vi "IMA Check Stop DC.vi"(0 "WFDC Notifier":refnum<notifier>, 7 "WFDC External Sync":refnum<notifier>, 11 "Error":errorcluster) -> (4 "WFDC Notifier (Dup)":refnum<notifier>, 8 "WFDC External Sync (Dup)":refnum<notifier>, 15 "Error Out":errorcluster)   [LabVIEW 2020]
uses:
  Wide Field Drift Correction/WFDC Controls/WFDC External Sync.ctl
  Wide Field Drift Correction/WFDC Controls/WFDC Cycle Pause.ctl
  Wide Field Drift Correction/WFDC Controls/WFDC Status.ctl
  Wide Field Drift Correction/WFDC Controls/WFDC Notifier Element.ctl
  Wide Field Drift Correction/WFDC Controls/WFDC Actions.ctl
  <vilib>/vision/Image Controls.llb/IMAQ Image.ctl
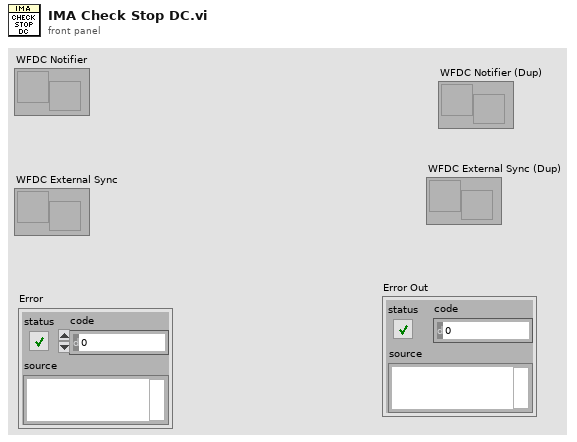
[diagram p1: front panel]
types:
  T1 = typedef "WFDC External Sync.ctl" = cluster{"Cycle Sync":T2, "Z Offset":dbl, "WFDC Status":T3}
  T2 = typedef "WFDC Cycle Pause.ctl" = enum16{"Pause Requested", "Paused", "Resume Requested", "Resumed"}
  T3 = typedef "WFDC Status.ctl" = enum16{"Idle", "Busy", "DC Active", "Error", "Canceled"}
  T4 = typedef "WFDC Notifier Element.ctl" = cluster{"WFDC Actions":T5, "Initial XYZ Positions":dbl[], "Ref Images":T6[], "Calibration (slope, inter)":dbl[], "Base Path":path, "Latest Scan Path":path, "Error":errorcluster, "XYZ Drift":dbl[]}
  T5 = typedef "WFDC Actions.ctl" = enum16{"Error Check", "Remote Start", "Move to Pos", "Pre Start Get Drift", "Pre Start Check Drift", "Pre Start Z Drift", "Pre Start XY Drift", "Pre Start ReFocus", "Setup New DC", "Setup Camera", "Get Ref Images", "Calc Calibration", "Switch Tabs", "Get Drift", "Z Drift", "XY Drift", "Start Cycle", "Stop DC", "Abort Remote", "Exit Loop", "Set Error", "Generate Calibration", "Quit"}
  T6 = typedef "IMAQ Image.ctl" = refnum<image>
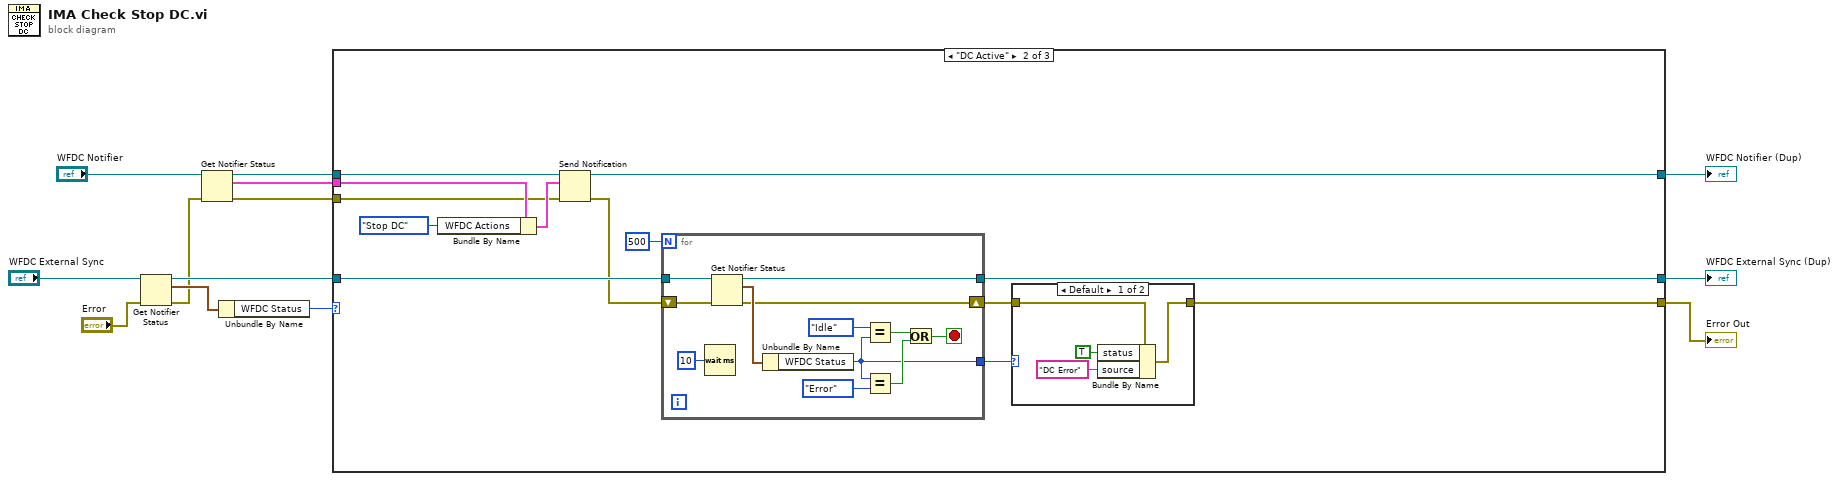
[diagram p0: block diagram]
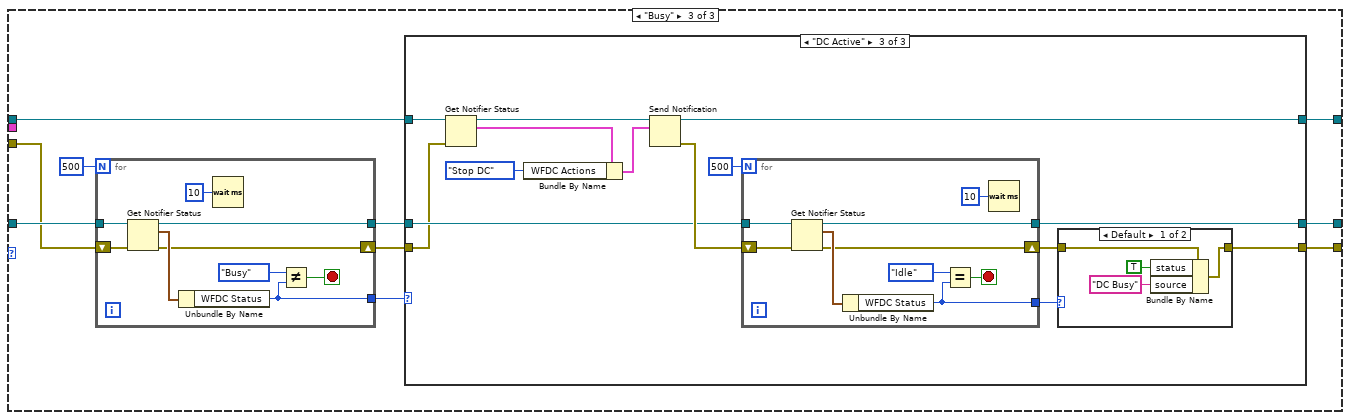
[diagram p4: hidden frame]
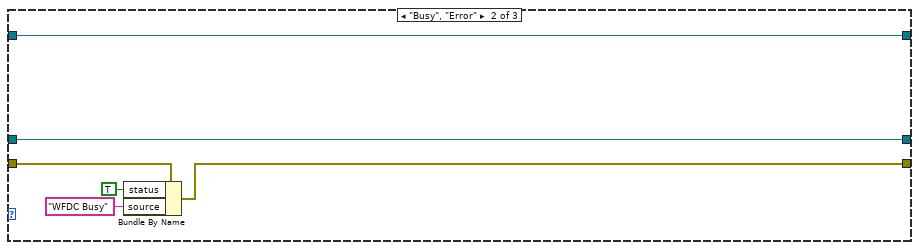
[diagram p6: hidden frame]
diagram:
  n1 = Get Notifier Status(notifier="WFDC External Sync", error in (no error)="Error") -> (notifier out=w13:refnum<notifier>, current notification=w12:T1, error out=w5:errorcluster)  [unwired: 2 out]
  n2 = Get Notifier Status(notifier="WFDC Notifier", error in (no error)=w5) -> (notifier out=w8:refnum<notifier>, current notification=w7:T4, error out=w6:errorcluster)  [unwired: 2 out]
  n3 = Unbundle By Name(w12) -> ("WFDC Status"=w11:T3)
  n4 = case shown="\"DC Active\"" w11 {
    tunnel: w13 -> [w15 w25 w56]
    tunnel: w8 -> [w16 w24 w49]
    tunnel: w7 -> [_ w27 _]
    tunnel: [w16 w26 w48] -> w1
    tunnel: [w15 w21 w51] -> w2
    tunnel: w6 -> [w14 w23 w55]
    tunnel: [w14 w17 w50] -> w3
    frame Default {
    }
    frame "DC Active" {
      n5 = Bundle By Name(cluster=w27, "WFDC Actions"=WFDC_Actions."Stop DC") -> (w28:T4)
      n6 = Send Notification(notification=w28, notifier=w24, error in (no error)=w23) -> (notifier out=w26:refnum<notifier>, error out=w22:errorcluster)
      n7 = for {
        N: 500 -> [_]
        tunnel: w25 -> [w45]
        tunnel: [w43] -> w21
        shift-right: [w41] -> w18
        shift-left: w22 -> [w42]
        tunnel: [w35] -> w19
        stop <- w36 stop-if-true
        n8 = Wait (ms)(milliseconds to wait=u32 10) -> ()  [unwired: 1 out]
        n9 = Get Notifier Status(notifier=w45, error in (no error)=w42) -> (notifier out=w43:refnum<notifier>, current notification=w46:T1, error out=w41:errorcluster)  [unwired: 2 out]
        n10 = Unbundle By Name(w46) -> ("WFDC Status"=w35:T3)
        n11 = Equal?(x=WFDC_Status."Idle", y=w35) -> (x = y?=w38:bool)
        n12 = Equal?(x=w35, y=WFDC_Status."Error") -> (x = y?=w37:bool)
        n13 = Or(x=w38, y=w37) -> (x .or. y?=w36:bool)
      }
      n14 = case shown="Default" w19 {
        tunnel: w18 -> [w33 w34]
        tunnel: [w30 w34] -> w17
        frame Default {
          n15 = Bundle By Name(cluster=w33, "status"=TRUE, "source"="DC Error") -> (w30:errorcluster)
        }
        frame "Idle", "Error" {
        }
      }
    }
    frame "Busy" {
      n16 = for {
        N: 500 -> [_]
        tunnel: w56 -> [w64]
        tunnel: [w62] -> w53
        shift-right: [w60] -> w52
        shift-left: w55 -> [w61]
        tunnel: [w58] -> w54
        stop <- w57 stop-if-true
        n17 = Get Notifier Status(notifier=w64, error in (no error)=w61) -> (notifier out=w62:refnum<notifier>, current notification=w65:T1, error out=w60:errorcluster)  [unwired: 2 out]
        n18 = Unbundle By Name(w65) -> ("WFDC Status"=w58:T3)
        n19 = Wait (ms)(milliseconds to wait=u32 10) -> ()  [unwired: 1 out]
        n20 = Not Equal?(x=WFDC_Status."Busy", y=w58) -> (x != y?=w57:bool)
      }
      n21 = case shown="\"DC Active\"" w54 {
        tunnel: w53 -> [w68 w73 w85]
        tunnel: w52 -> [w67 w72 w79]
        tunnel: [w68 w73 w84] -> w51
        tunnel: [w67 w69 w75] -> w50
        tunnel: [w66 w74 w83] -> w48
        tunnel: w49 -> [w66 w74 w82]
        frame Default {
        }
        frame "Busy", "Error" {
          n22 = Bundle By Name(cluster=w72, "status"=TRUE, "source"="WFDC Busy") -> (w69:errorcluster)
        }
        frame "DC Active" {
          n23 = Get Notifier Status(notifier=w82, error in (no error)=w79) -> (notifier out=w81:refnum<notifier>, current notification=w80:T4)  [unwired: 3 out]
          n24 = Bundle By Name(cluster=w80, "WFDC Actions"=WFDC_Actions."Stop DC") -> (w87:T4)
          n25 = Send Notification(notification=w87, notifier=w81) -> (notifier out=w83:refnum<notifier>, error out=w86:errorcluster)  [unwired: 1 in]
          n26 = for {
            N: 500 -> [_]
            tunnel: w85 -> [w101]
            tunnel: [w99] -> w84
            shift-right: [w97] -> w76
            shift-left: w86 -> [w98]
            tunnel: [w94] -> w77
            stop <- w95 stop-if-true
            n27 = Get Notifier Status(notifier=w101, error in (no error)=w98) -> (notifier out=w99:refnum<notifier>, current notification=w102:T1, error out=w97:errorcluster)  [unwired: 2 out]
            n28 = Unbundle By Name(w102) -> ("WFDC Status"=w94:T3)
            n29 = Equal?(x=WFDC_Status."Idle", y=w94) -> (x = y?=w95:bool)
            n30 = Wait (ms)(milliseconds to wait=u32 10) -> ()  [unwired: 1 out]
          }
          n31 = case shown="Default" w77 {
            tunnel: w76 -> [w92 w93]
            tunnel: [w90 w93] -> w75
            frame Default {
              n32 = Bundle By Name(cluster=w92, "status"=TRUE, "source"="DC Busy") -> (w90:errorcluster)
            }
            frame "Idle" {
            }
          }
        }
      }
    }
  }
  "Error Out" <- w3
  "WFDC External Sync (Dup)" <- w2
  "WFDC Notifier (Dup)" <- w1
